vi "SRV_VIG_System Config Name.vi"(6 "Method (Get)":enum16{"Get", "Set"}(ring), 8 "error in (no error)":errorcluster, 9 "SystemConfig Filepath":path, 10 "System Config Name":string) -> (0 "error out":errorcluster, 1 "SystemConfig Filepath out":path, 2 "System Config Name out":string)   [LabVIEW 2014]
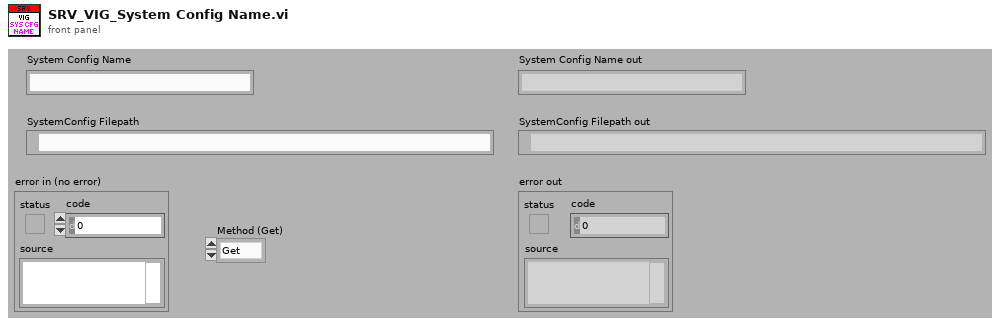
[diagram p1: front panel]
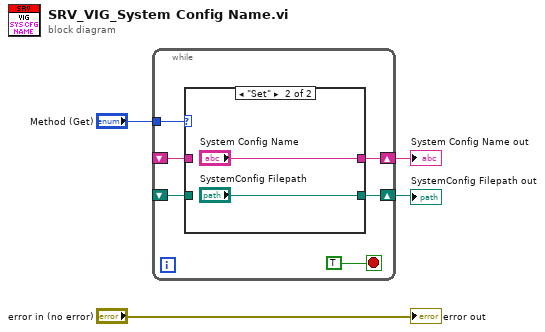
[diagram p0: block diagram]
diagram:
  n1 = while {
    tunnel: "Method (Get)" -> [w10]
    shift-right: [w8] -> w2
    shift-left: _ -> [w9]
    shift-right: [w6] -> w1
    shift-left: _ -> [w5]
    stop <- TRUE stop-if-true
    n2 = case shown="\"Set\"" w10 {
      tunnel: w9 -> [w12 _]
      tunnel: [w12 "System Config Name"] -> w8
      tunnel: [w11 "SystemConfig Filepath"] -> w6
      tunnel: w5 -> [w11 _]
      frame "Get" {
      }
      frame "Set" {
      }
    }
  }
  "System Config Name out" <- w2
  "SystemConfig Filepath out" <- w1
  "error out" <- "error in (no error)"
